vi "RandomLaser20.vi"() -> ()   [LabVIEW 2021]
doc: "Random Laser Project v2.0\nAndré Romero - 2024\nandretec@ifsc.usp.br"
uses:
  State-MainLoop.ctl
  Global_v20.vi
panel:
  in  "Tab Control":T1(tab)
  in  "Simulation mode":bool=TRUE
  in  "Average":i32=1
  in  "Integration Time (ms)":i32=100
  out "Spectrum":T2(graph)
  in  "Store Dark Spec":bool caption="Blank Button"
  in  "Clear Dark Spec":bool caption="Blank Button"
  out "Power Meter (W)":dbl=1.0400848399440292 format="%#_4p"
  out "Power Graph":dbl[](graph)=[1.2567462692095432, 1.2371684292156715, 1.22313764388673, 1.2120435345568694, 1.2032335065596271, 1.1937708838959225, 1.1816978825663682, 1.172887854569126, 1.1588570692401845, 1.1451525812444743, 1.1353636612475384, 1.1232906599179842, 1.1082809825893492, 1.104691711923806, 1.0971868732594885, 1.0900083319284022, 1.0893557372619398, 1.0860927639296278, 1.0834823852637783, 1.0769564385991544, 1.0743460599333048, 1.0769564385991544, 1.0710830866009928, 1.0691253026016057, 1.076303843932692, 1.0769564385991544, 1.0727145732671488, 1.0740197626000736, 1.069777897268068, 1.0521578412735835, 1.047915975941578, 1.0583574906049762, 1.076303843932692, 1.0821771959308535, 1.0821771959308535, 1.0834823852637783, 1.0851138719299342, 1.0736934652668424, 1.0639045452699065, 1.0400848399440292]
  in  "Average Time (sec)":dbl=0.1 caption="Average Time (0.0)"
  in  "StepperMotor":bool
  out "Steps Chart":dbl(graph)=0.008999878500492074
  out "Current Step":i32=110
  in  "Play Aquisition":bool
  in  "Save Aquisition":bool
  out "FWHM":cluster{dbl[], dbl[]}(graph)={[0.012126, 0.012384, 0.012641999999999999, 0.012899999999999998, 0.013158, 0.013415999999999999, 0.013673999999999999, 0.013932, 0.01419, 0.014447999999999999, 0.014705999999999999, 0.014963999999999998, 0.015222, 0.015479999999999999, 0.015738, 0.015996, 0.016253999999999998, 0.016512, 0.01677, 0.017027999999999998, 0.017286, 0.017543999999999997, 0.017802, 0.01806, 0.018317999999999997, 0.018576, 0.018834, 0.019091999999999998, 0.01935, 0.019608, 0.019865999999999998, 0.020124, 0.020381999999999997, 0.02064, 0.020898, 0.021155999999999998, 0.021414, 0.021671999999999997, 0.021929999999999998, 0.022188, 0.022445999999999997, 0.022704, 0.022962, 0.023219999999999998, 0.023478, 0.023736, 0.023993999999999998, 0.024252, 0.024509999999999997], [563.31395, 575.661165, 575.661165, 528.932198, 670.156069, 604.385078, 636.3367910000001, 511.96710499999995, 504.872479, 67.578758, 68.90254600000003, 67.20192599999996, 63.7958329999999, 57.57778500000006, 53.10652100000004, 48.27215699999999, 45.172767999999905, 43.09348499999999, 40.679044999999974, 56.891447000000085, 38.94813799999997, 38.262392999999975, 37.90251999999998, 36.170840999999996, 34.44723299999998, 34.44723299999998, 35.138649999999984, 34.792963999999984, 34.792963999999984, 33.05966699999999, 30.637351999999964, 29.948648999999932, 29.598544999999945, 24.045388000000003, 24.045388000000003, 24.045388000000003, 26.823037, 27.86278200000004, 25.779633999999987, 21.962823999999955, 21.615575000000035, 19.87615900000003, 19.87615900000003, 17.440737000000013, 18.48600799999997, 17.790666999999985, 17.790666999999985, 18.136077999999998, 17.095147999999995]}
  out "PEAK":cluster{dbl[], dbl[]}(graph)={[0.012126, 0.012384, 0.012641999999999999, 0.012899999999999998, 0.013158, 0.013415999999999999, 0.013673999999999999, 0.013932, 0.01419, 0.014447999999999999, 0.014705999999999999, 0.014963999999999998, 0.015222, 0.015479999999999999, 0.015738, 0.015996, 0.016253999999999998, 0.016512, 0.01677, 0.017027999999999998, 0.017286, 0.017543999999999997, 0.017802, 0.01806, 0.018317999999999997, 0.018576, 0.018834, 0.019091999999999998, 0.01935, 0.019608, 0.019865999999999998, 0.020124, 0.020381999999999997, 0.02064, 0.020898, 0.021155999999999998, 0.021414, 0.021671999999999997, 0.021929999999999998, 0.022188, 0.022445999999999997, 0.022704, 0.022962, 0.023219999999999998, 0.023478, 0.023736, 0.023993999999999998, 0.024252, 0.024509999999999997], [1087.395556, 1179.63, 1179.63, 1203.902222, 1196.620556, 1320.408889, 1504.877778, 1691.773889, 1716.046111, 2206.345, 2364.114444, 2402.95, 2497.611667, 2657.808333, 3026.746111, 3361.702778, 3779.185, 4009.771111, 4133.559444, 2623.827222, 4604.440556, 4711.238333, 5102.021111, 5543.775556, 5924.849444, 5924.849444, 6111.745556, 6063.201111, 6063.201111, 7216.131667, 7810.801111, 8383.625556, 7966.143333, 11546.296111, 11546.296111, 11822.999444, 10082.681111, 9342.378333, 10995.316667, 15417.715556, 15347.326111, 16917.738889, 16917.738889, 20437.211111, 19604.673889, 21410.527222, 20352.258333, 20245.460556, 21199.358889]}
  out "Signal":T2(graph)
  in  "Total points":i32=49
  in  "Stop":bool
  in  "min Power":bool
  in  "max Power":bool
  out "Power Meter [W]":dbl=0.0009074480409090909 format="%#_4p"
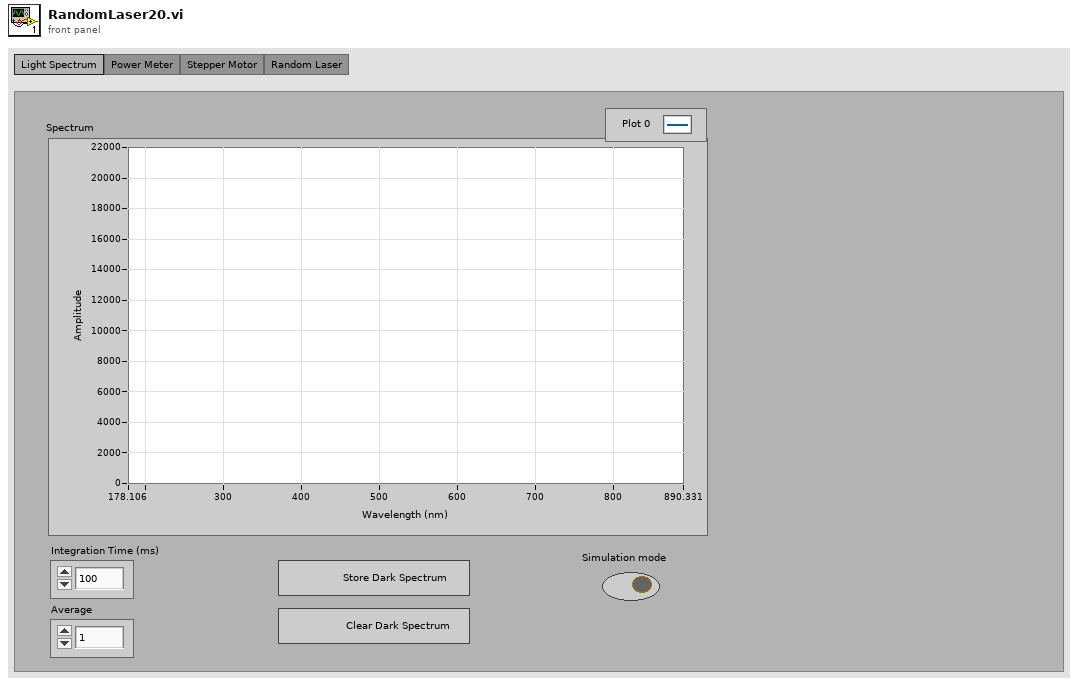
[diagram p1: front panel]
types:
  T1 = enum32{"Light Spectrum", "Power Meter", "Stepper Motor", "Random Laser"}
  T2 = cluster{"WL Values":dbl[], "Spectrum Values":dbl[]}
  T3 = typedef "State-MainLoop.ctl" = enum16{"Initialize", "Wait for Event", "Spectrum Graph", "Power Meter", "Stepper Motor", "Random Laser"}
  T4 = enum8{"Enabled", "Disabled", "Disabled and Grayed Out"}
  T5 = enum32{"Page Enabled", "Page Disabled", "Page Disabled & Grayed"}
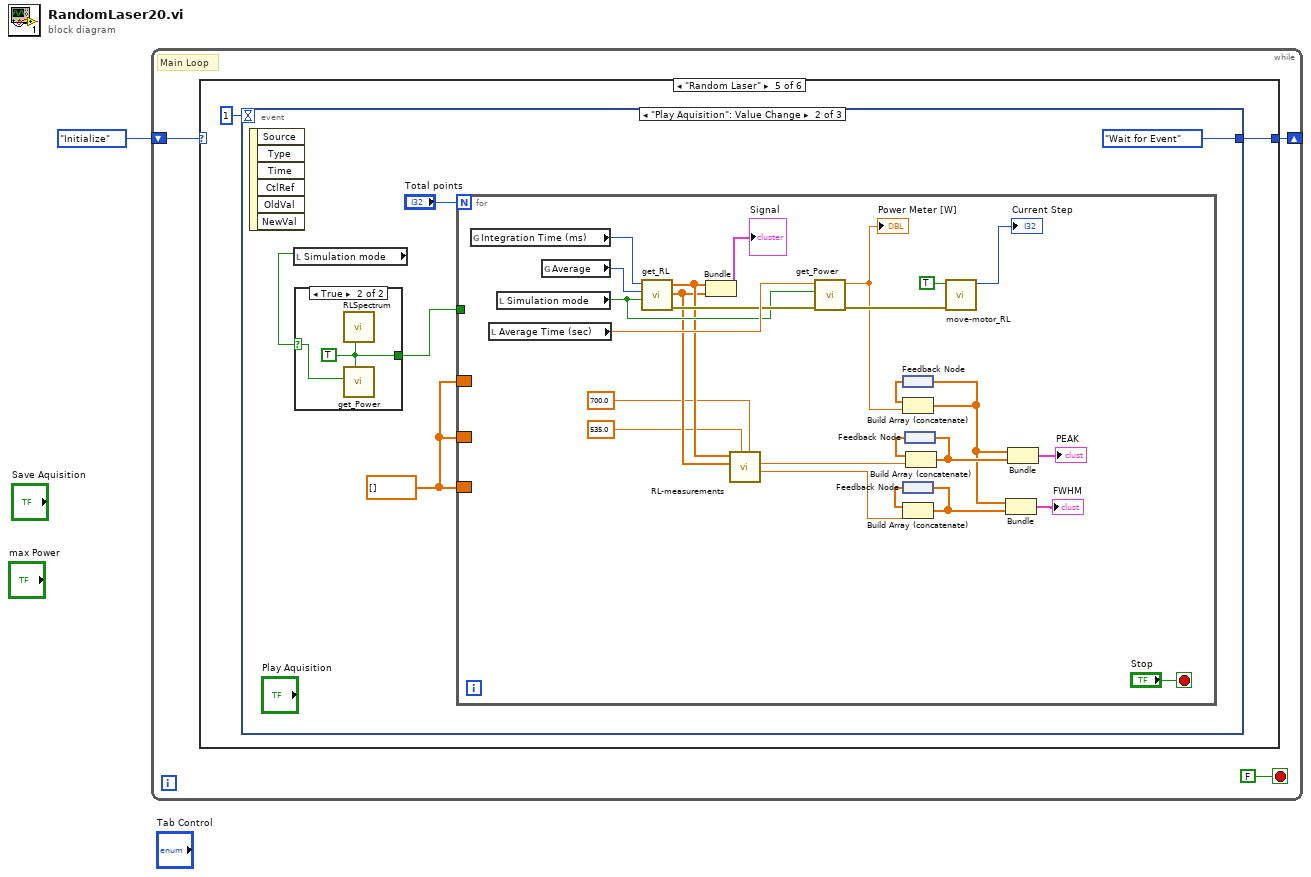
[diagram p0: block diagram]
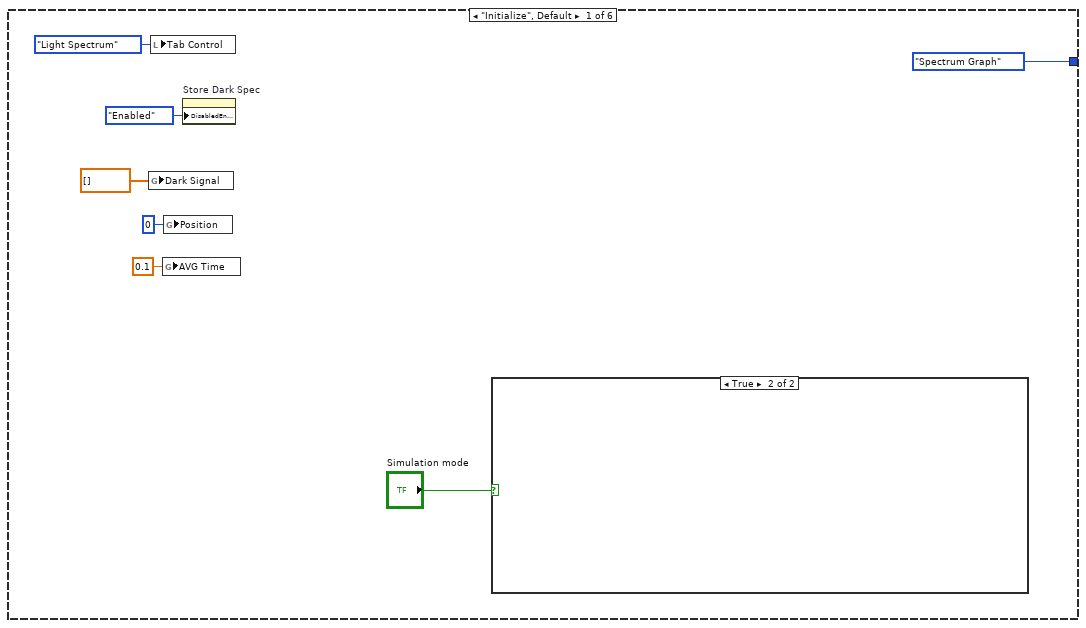
[diagram p2: hidden frame]
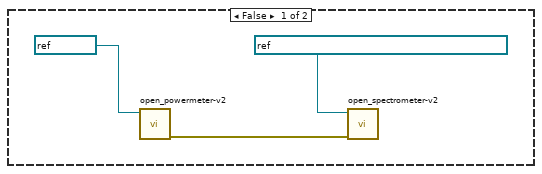
[diagram p3: hidden frame]
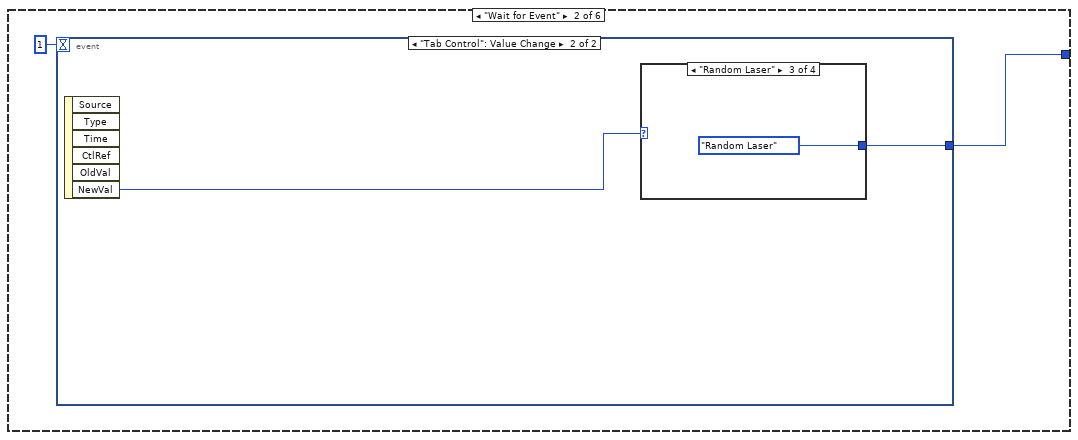
[diagram p4: hidden frame]
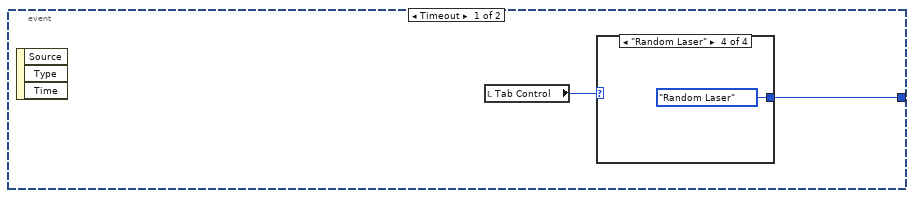
[diagram p5: hidden frame]
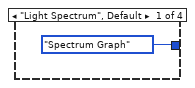
[diagram p6: hidden frame]
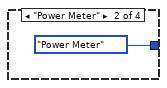
[diagram p7: hidden frame]
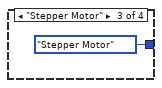
[diagram p8: hidden frame]
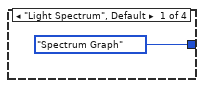
[diagram p9: hidden frame]
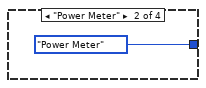
[diagram p10: hidden frame]
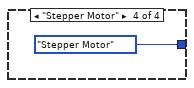
[diagram p11: hidden frame]
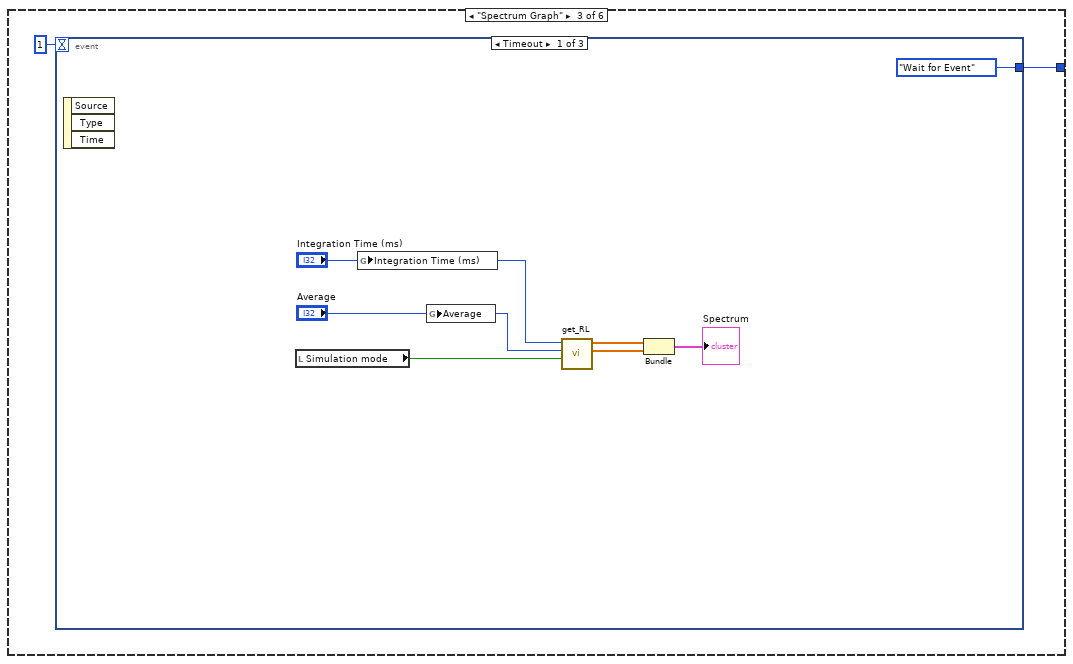
[diagram p12: hidden frame]
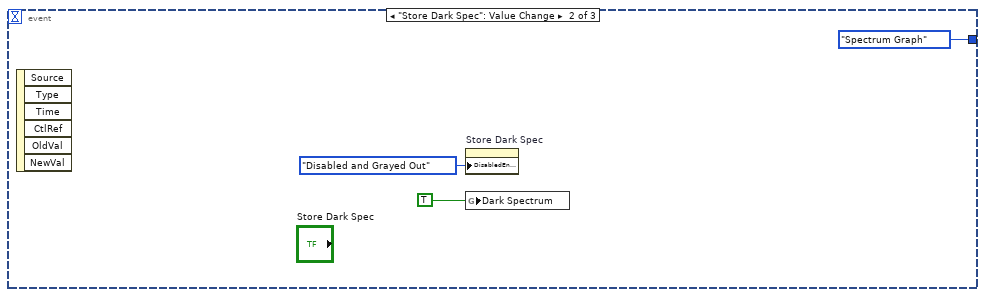
[diagram p13: hidden frame]
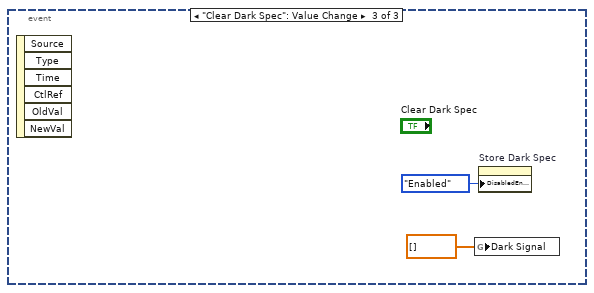
[diagram p14: hidden frame]
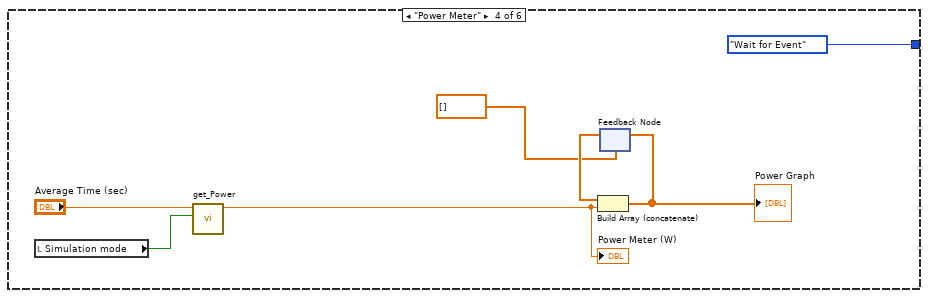
[diagram p15: hidden frame]
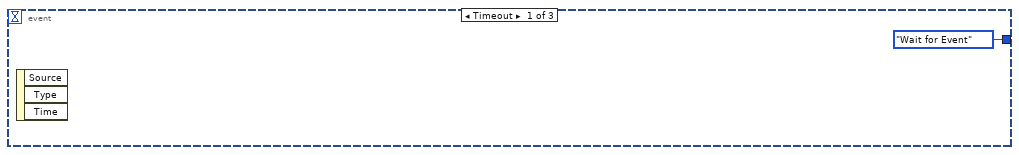
[diagram p16: hidden frame]
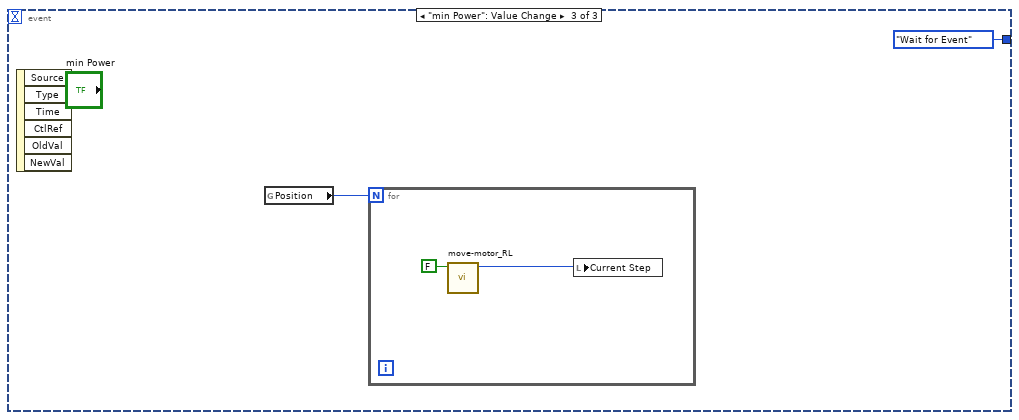
[diagram p18: hidden frame]
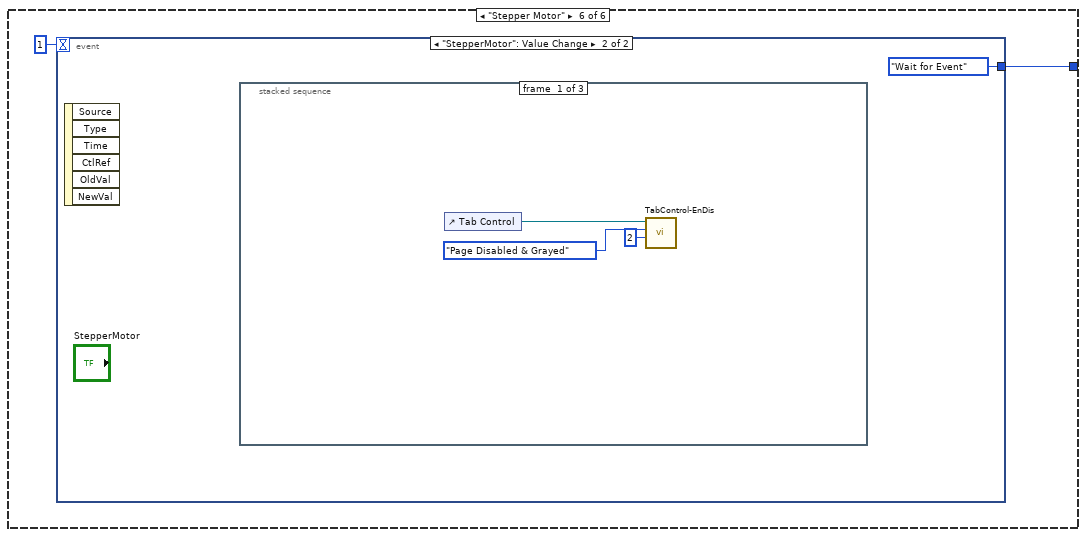
[diagram p19: hidden frame]
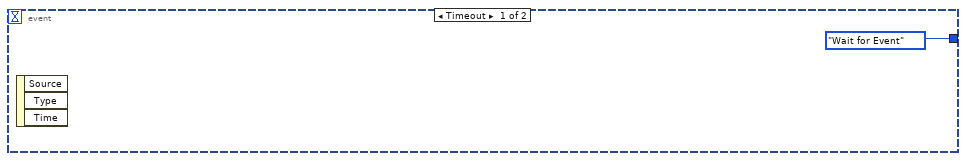
[diagram p20: hidden frame]
diagram:
  n1 = while {
    shift-right: [w2] -> _
    shift-left: State-MainLoop."Initialize" -> [w3]
    stop <- FALSE stop-if-true
    # "Main Loop"
    n2 = case shown="\"Random Laser\"" w3 {
      tunnel: [State-MainLoop."Spectrum Graph" w16 w30 State-MainLoop."Wait for Event" w51 w89] -> w2
      frame "Initialize", Default {
        n3 = global write "Global_v20.vi" "Dark Signal"(dbl[] []) -> ()
        n4 = local write "Tab Control"(T1."Light Spectrum" ("Tab Control")) -> ()
        n5 = global write "Global_v20.vi" "AVG Time"(0.1 ("AVG Time")) -> ()
        n6 = global write "Global_v20.vi" "Position"(0 ("Position")) -> ()
        n7 = property on="Store Dark Spec" class="Bool"("DisabledEnum"=T4."Enabled" ("Disabled")) -> ()  [unwired: 2 in, 2 out]
        n8 = case shown="True" "Simulation mode" {
          frame False {
            n9 = call "open_powermeter-v2.vi"("VISA Refnum in"=refnum<visa-resource-name> "COM3" ("instrument handle")) -> ("error out"=w13:errorcluster)  [unwired: 10 in]
            n10 = call "open_spectrometer-v2.vi"("error in"=w13, "VISA Refnum in"=refnum<visa-resource-name> "USB0::0x2457::0x101E::NI-VISA-40002::RAW" ("VISA resource name")) -> ()  [unwired: 8 in, 2 out]
          }
          frame True {
          }
        }
      }
      frame "Wait for Event" {
        n11 = event shown="[1] \"Tab Control\": Value Change" {
          selector: _ -> [_ _]
          dyn-events: _ -> [_ _]
          timeout: 1 -> [_ _]
          tunnel: [w18 w23] -> w16
          event Timeout {
            n12 = event-data() -> ()  [unwired: 1 in, 3 out]
            n13 = local read "Tab Control"() -> (w17:T1)
            n14 = case shown="\"Random Laser\"" w17 {
              tunnel: [State-MainLoop."Spectrum Graph" State-MainLoop."Power Meter" State-MainLoop."Stepper Motor" State-MainLoop."Random Laser"] -> w18
              frame "Light Spectrum", Default {
              }
              frame "Power Meter" {
              }
              frame "Stepper Motor" {
              }
              frame "Random Laser" {
              }
            }
          }
          event "Tab Control": Value Change {
            n15 = event-data() -> ("NewVal"=w24:T1)  [unwired: 1 in, 5 out]
            n16 = case shown="\"Random Laser\"" w24 {
              tunnel: [State-MainLoop."Spectrum Graph" State-MainLoop."Power Meter" State-MainLoop."Random Laser" State-MainLoop."Stepper Motor"] -> w23
              frame "Light Spectrum", Default {
              }
              frame "Power Meter" {
              }
              frame "Random Laser" {
              }
              frame "Stepper Motor" {
              }
            }
          }
        }
      }
      frame "Spectrum Graph" {
        n17 = event shown="[0] Timeout" {
          selector: _ -> [_ _ _]
          dyn-events: _ -> [_ _ _]
          timeout: 1 -> [_ _ _]
          tunnel: [State-MainLoop."Wait for Event" State-MainLoop."Spectrum Graph" _] -> w30
          event Timeout {
            n18 = event-data() -> ()  [unwired: 1 in, 3 out]
            n19 = local read "Simulation mode"() -> (w34:bool)
            n20 = global write "Global_v20.vi" "Integration Time (ms)"("Integration Time (ms)") -> ()
            n21 = global write "Global_v20.vi" "Average"("Average") -> ()
            n22 = call "get_RL.vi"("Simulation mode"=w34, "Average"="Average", "Integration Time (ms)"="Integration Time (ms)") -> ("RL Spectrum"=w33:dbl[], "WL Values"=w35:dbl[])  [unwired: 6 in, 1 out]
            n23 = Bundle("WL Values"=w35, "RL Spectrum"=w33) -> (→"Spectrum":cluster{"WL Values":dbl[], "RL Spectrum":dbl[]})  [unwired: 1 in]
          }
          event "Store Dark Spec": Value Change {
            n24 = event-data() -> ()  [unwired: 1 in, 6 out]
            n25 = property on="Store Dark Spec" class="Bool"("DisabledEnum"=T4."Disabled and Grayed Out" ("Disabled")) -> ()  [unwired: 2 in, 2 out]
            n26 = global write "Global_v20.vi" "Dark Spectrum"(TRUE ("Dark Spec")) -> ()
          }
          event "Clear Dark Spec": Value Change {
            n27 = event-data() -> ()  [unwired: 1 in, 6 out]
            n28 = global write "Global_v20.vi" "Dark Signal"(dbl[] []) -> ()
            n29 = property on="Store Dark Spec" class="Bool"("DisabledEnum"=T4."Enabled" ("Disabled")) -> ()  [unwired: 2 in, 2 out]
          }
        }
      }
      frame "Power Meter" {
        n30 = local read "Simulation mode"() -> (w46:bool)
        n31 = call "get_Power.vi"("Simulation mode"=w46, "Average Time (sec)"="Average Time (sec)") -> ("Power"=w45:dbl)  [unwired: 8 in, 1 out]
        "Power Meter (W)" <- w45
        n32 = feedback #1(dbl[] []) -> (w48:dbl[])
        n33 = Build Array (concatenate)(w48, w45) -> (w47:dbl[])
        "Power Graph" <- w47
        n34 = feedback-in #1(w47) -> ()
      }
      frame "Random Laser" {
        n35 = event shown="[1] \"Play Aquisition\": Value Change" {
          selector: _ -> [_ _ _]
          dyn-events: _ -> [_ _ _]
          timeout: 1 -> [_ _ _]
          tunnel: [State-MainLoop."Wait for Event" State-MainLoop."Wait for Event" State-MainLoop."Wait for Event"] -> w51
          event Timeout {
            n36 = event-data() -> ()  [unwired: 1 in, 3 out]
          }
          event "Play Aquisition": Value Change {
            w53 = dbl[] []
            n37 = event-data() -> ()  [unwired: 1 in, 6 out]
            n38 = local read "Simulation mode"() -> (w54:bool)
            n39 = case shown="True" w54 {
              selector: w54 -> [_ w58]
              tunnel: [_ w59] -> w55
              frame False {
              }
              frame True {
                w59 = TRUE ("reset")
                n40 = call "RLSpectrum.vi"("reset"=w59) -> ()  [unwired: 9 in, 2 out]
                n41 = call "get_Power.vi"("reset"=w59, "Simulation mode"=w58) -> ()  [unwired: 8 in, 2 out]
              }
            }
            n42 = for {
              N: "Total points" -> [_]
              tunnel: w55 -> [_]
              border: w53 -> [_]
              border: w53 -> [_]
              border: w53 -> [_]
              stop <- "Stop" stop-if-true
              n43 = global read "Global_v20.vi" "Integration Time (ms)"() -> (w83:i32)
              n44 = local read "Average Time (sec)"() -> (w80:dbl)
              n45 = local read "Simulation mode"() -> (w75:bool)
              n46 = global read "Global_v20.vi" "Average"() -> (w82:i32)
              n47 = call "get_RL.vi"("Simulation mode"=w75, "Average"=w82, "Integration Time (ms)"=w83) -> ("error out"=w79:errorcluster, "RL Spectrum"=w73:dbl[], "WL Values"=w74:dbl[])  [unwired: 6 in]
              n48 = Bundle("WL Values"=w74, "RL Spectrum"=w73) -> (→"Signal":cluster{"WL Values":dbl[], "RL Spectrum":dbl[]})  [unwired: 1 in]
              n49 = call "RL-measurements.vi"("WL final"=700.0, "WL initial"=535.0, "RL Spectrum"=w73, "WL Values"=w74) -> ("FWHM"=w68:dbl, "Peak value"=w60:dbl)  [unwired: 2 in, 3 out]
              n50 = call "get_Power.vi"("error in"=w79, "Simulation mode"=w75, "Average Time (sec)"=w80) -> ("error out"=w76:errorcluster, "Power"=w66:dbl)  [unwired: 7 in]
              "Power Meter [W]" <- w66
              n51 = feedback #2() -> (w67:dbl[])
              n52 = Build Array (concatenate)(w67, w66) -> (w62:dbl[])
              n53 = feedback-in #2(w62) -> ()
              n54 = feedback #3() -> (w69:dbl[])
              n55 = Build Array (concatenate)(w69, w68) -> (w65:dbl[])
              n56 = feedback-in #3(w65) -> ()
              n57 = feedback #4() -> (w70:dbl[])
              n58 = Build Array (concatenate)(w70, w60) -> (w63:dbl[])
              n59 = feedback-in #4(w63) -> ()
              n60 = call "move-motor_RL.vi"("error in"=w76, "Direction"=TRUE) -> ("Current Stepp"=→"Current Step":i32)  [unwired: 8 in, 1 out]
              n61 = Bundle(w62, w65) -> (→"FWHM":cluster{dbl[], dbl[]})  [unwired: 1 in]
              n62 = Bundle(w62, w63) -> (→"PEAK":cluster{dbl[], dbl[]})  [unwired: 1 in]
            }
          }
          event "min Power": Value Change {
            n63 = event-data() -> ()  [unwired: 1 in, 6 out]
            n64 = global read "Global_v20.vi" "Position"() -> (w86:i32)
            n65 = for {
              N: w86 -> [_]
              n66 = call "move-motor_RL.vi"("Direction"=FALSE) -> ("Current Stepp"=w87:i32)  [unwired: 9 in, 1 out]
              n67 = local write "Current Step"(w87) -> ()
            }
          }
        }
      }
      frame "Stepper Motor" {
        n68 = event shown="[1] \"StepperMotor\": Value Change" {
          selector: _ -> [_ _]
          dyn-events: _ -> [_ _]
          timeout: 1 -> [_ _]
          tunnel: [State-MainLoop."Wait for Event" State-MainLoop."Wait for Event"] -> w89
          event Timeout {
            n69 = event-data() -> ()  [unwired: 1 in, 3 out]
          }
          event "StepperMotor": Value Change {
            n70 = event-data() -> ()  [unwired: 1 in, 6 out]
            n71 = stacked-sequence {
              frame #0 {
                n72 = control-ref of="Tab Control"() -> (w94:refnum<vi>)
                n73 = call "TabControl-EnDis.vi"("Tab"=2, "Tab Enabled State"=T5."Page Disabled & Grayed" ("Page Enabled State"), "TabControl in"=w94) -> ()  [unwired: 8 in, 1 out]
              }
              frame #1 {
                n74 = for {
                  N: 10 -> [_]
                  i -> [w101]
                  n75 = Divide(x=w101, y=1000) -> (x/y=w99:dbl)
                  n76 = Sine(x=w99) -> (sin(x)=→"Steps Chart":dbl)
                  n77 = Wait (ms)(milliseconds to wait=u32 500) -> ()  [unwired: 1 out]
                }
              }
              frame #2 {
                n78 = control-ref of="Tab Control"() -> (w103:refnum<vi>)
                n79 = call "TabControl-EnDis.vi"("Tab"=2 ("Page"), "Tab Enabled State"=T5."Page Enabled" ("Page Enabled State"), "TabControl in"=w103) -> ()  [unwired: 8 in, 1 out]
              }
            }
          }
        }
      }
    }
  }
